vi "1D-Array_Mean_SD_EXAMPLE.vi"() -> ()   [LabVIEW 2013]
panel:
  in  "stop":bool
  out "Standard Deviation":dbl[](array[numeric])
  out "Mean":dbl[](array[numeric])
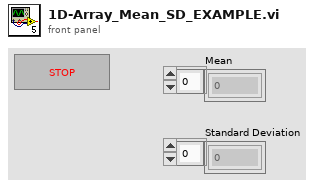
[diagram p1: front panel]
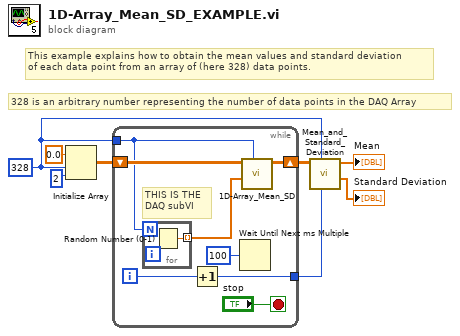
[diagram p0: block diagram]
diagram:
  w1 = 328 ("dimension size")
  # "This example explains how to obtain the mean values and standard deviation\nof each data point from an array of (here 328) data points."
  # "328 is an arbitrary number representing the number of data points in the DAQ Array"
  n1 = Initialize Array(0.0 ("element"), w1, 2 ("dimension size")) -> (w6:dbl[][])
  n2 = while {
    tunnel: w1 -> [w12]
    shift-right: [w15] -> w5
    shift-left: w6 -> [w16]
    tunnel: [w13] -> w4
    i -> [w14]
    stop <- "stop" stop-if-true
    # "THIS IS THE \nDAQ subVI"
    n3 = for {
      N: w12 -> [_]
      tunnel: [w17] -> w10 mode=indexing
      n4 = Random Number (0-1)() -> (number: 0 to 1=w17:dbl)
    }
    n5 = Increment(x=w14) -> (x+1=w13:i32)
    n6 = Wait Until Next ms Multiple(millisecond multiple=u32 100) -> ()  [unwired: 1 out]
    n7 = call "1D-Array_Mean_SD.vi"("N"=w12, "Data Array"=w10, "IN"=w16) -> ("OUT"=w15:dbl[][])  [unwired: 8 in]
  }
  n8 = call "Mean_and_Standard_Deviation.vi"("Iterations"=w4, "Data Points"=w1, "2D array"=w5) -> ("Standard Deviation"=→"Standard Deviation":dbl[], "Mean"=→"Mean":dbl[])  [unwired: 7 in]
